vi "understanding looping array quotient.vi"() -> ()   [LabVIEW 2012]
panel:
  in  "Array":dbl[](array[numeric])
  in  "stop":bool
  out "x-y*floor(x/y) 2":i32
  out "x-y*floor(x/y)":i32
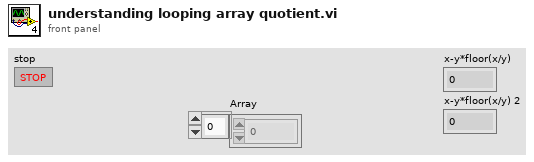
[diagram p1: front panel]
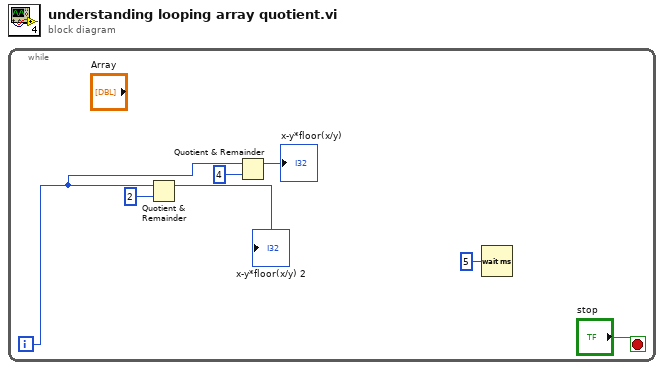
[diagram p0: block diagram]
diagram:
  n1 = while {
    i -> [w6]
    stop <- "stop" stop-if-true
    n2 = Quotient & Remainder(x=w6, y=2) -> (x-y*floor(x/y)=→"x-y*floor(x/y) 2":i32)  [unwired: 1 out]
    n3 = Quotient & Remainder(x=w6, y=4) -> (x-y*floor(x/y)=→"x-y*floor(x/y)":i32)  [unwired: 1 out]
    n4 = Wait (ms)(milliseconds to wait=u32 5) -> ()  [unwired: 1 out]
  }
